vi "Digital Output Update Data.vi"(4 "Main Engine Response Q":refnum<queue>, 6 "TCP Engine Response Q":refnum<queue>, 7 "Task in":refnum<k21>, 8 "error in":errorcluster, 9 "Path":path, 10 "Interupt Q":refnum<queue>, 11 "DO Config Data":T1) -> (0 "error out":errorcluster, 2 "Stop":bool, 3 "DO Config Data Out":T1)   [LabVIEW 2024]
doc: "All Rights Reserved © 2017 SyncSols"
uses:
  TCP Engine/Controls/TCP Engine I&O  Interupt Cluster.ctl
  Host-DQMH/Configuration/DO Channel's.ctl
  fdad0fac-ba06-49f9-8619-3fd954bcf845.vi
  <vilib>/DAQmx/write.llb/DAQmx Write (Digital 1D Bool NChan 1Samp 1Line).vi
  <vilib>/DAQmx/miscellaneous.llb/DAQmx Fill In Error Info.vi
  TCP Engine/TCP Engine.lvlib
  Host-DQMH/Configuration/Configuration.lvlib
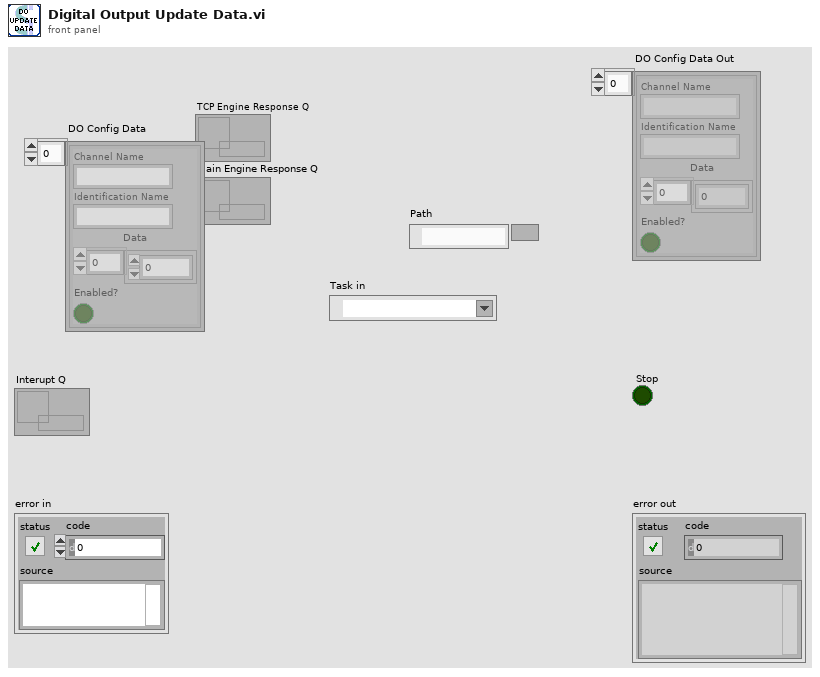
[diagram p1: front panel]
types:
  T1 = typedef "Configuration.lvlib/DO Channel's.ctl" = cluster{"Channel Name":string, "Identification Name":string, "Data":u8[], "Enabled?":bool}[]
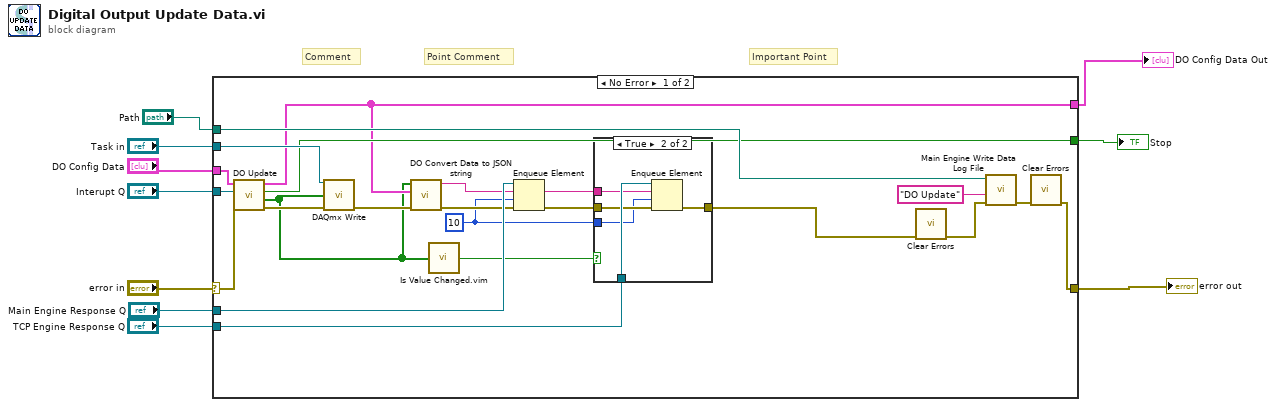
[diagram p0: block diagram]
diagram:
  # "Important Point"
  # "Point Comment"
  # "Comment"
  n1 = case shown="No Error" "error in" {
    selector: "error in" -> [w30 w40]
    tunnel: [w11 w40] -> w10
    tunnel: "Path" -> [w32 _]
    tunnel: "Task in" -> [w31 _]
    tunnel: "DO Config Data" -> [w28 w39]
    tunnel: [w24 w39] -> w2
    tunnel: "Interupt Q" -> [w27 _]
    tunnel: [w26 _] -> w6
    tunnel: "TCP Engine Response Q" -> [w23 _]
    tunnel: "Main Engine Response Q" -> [w22 _]
    frame No Error {
      w14 = 10 ("timeout in ms (-1)")
      n2 = call "DO Update.vi"("error in"=w30, "Interupt Q"=w27, "DO Config Data"=w28) -> ("error out"=w29:errorcluster, "Data to Generate"=w21:bool[], "Stop"=w26:bool, "DO Config Data 2"=w24:T1)  [unwired: 5 in]
      n3 = call-poly <vilib>:"DAQmx Write.vi"("task/channels in"=w31, "data"=w21, "error in"=w29) -> ("error out"=w25:errorcluster)  [unwired: 10 in, 2 out]
      n4 = call "DO Convert Data to JSON string.vi"("error in"=w25, "DO Config Data"=w24, "Data In"=w21) -> ("error out"=w16:errorcluster, "JSON String"=w17:string)  [unwired: 7 in]
      n5 = call "Is Value Changed.vim"("value"=w21) -> ("changed or first call?"=w13:bool)
      n6 = Enqueue Element(queue=w22, element=w17, timeout in ms (-1)=w14, error in (no error)=w16) -> (error out=w15:errorcluster)  [unwired: 2 out]
      n7 = case shown="True" w13 {
        tunnel: w23 -> [_ w38]
        tunnel: w17 -> [_ w37]
        tunnel: w15 -> [w33 w36]
        tunnel: w14 -> [_ w35]
        tunnel: [w33 w34] -> w12
        frame False {
        }
        frame True {
          n8 = Enqueue Element(queue=w38, element=w37, timeout in ms (-1)=w35, error in (no error)=w36) -> (error out=w34:errorcluster)  [unwired: 2 out]
        }
      }
      n9 = call <vilib>:"Clear Errors.vi"("error in (no error)"=w12) -> ("error out"=w18:errorcluster)  [unwired: 5 in, 1 out]
      n10 = call "Main Engine Write Data Log File.vi"("error in"=w18, "State"="DO Update", "Log file path In"=w32) -> ("error out"=w19:errorcluster)  [unwired: 7 in, 1 out]
      n11 = call <vilib>:"Clear Errors.vi"("error in (no error)"=w19) -> ("error out"=w11:errorcluster)  [unwired: 5 in, 1 out]
    }
    frame Error {
    }
  }
  "error out" <- w10
  "Stop" <- w6
  "DO Config Data Out" <- w2
